vi "LS218_INIT_VOIES.vi"(2 "Tableau 2":T1(array[cluster]), 7 "entrée d'erreur (pas d'erreur)":errorcluster, 10 "Refnum VISA en entrée":refnum<visa-resource-name>) -> (0 "error out":errorcluster, 3 "Refnum VISA en entrée 2":refnum<visa-resource-name>)   [LabVIEW 2014]
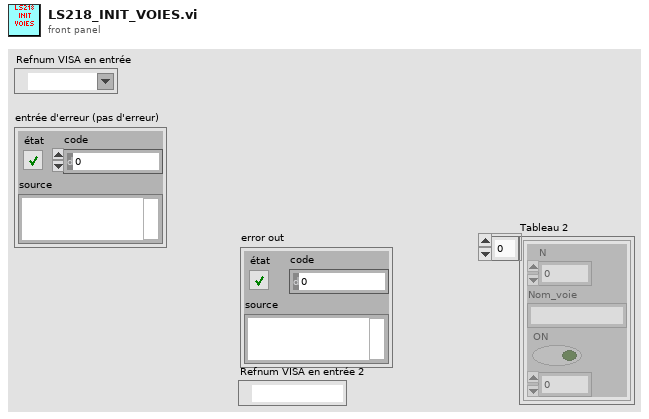
[diagram p1: front panel]
types:
  T1 = cluster{"N":i32, "Nom_voie":string, "ON":bool, dbl}[]
  T2 = cluster{"N":i32, "Nom_voie":string, "ON":bool, dbl}
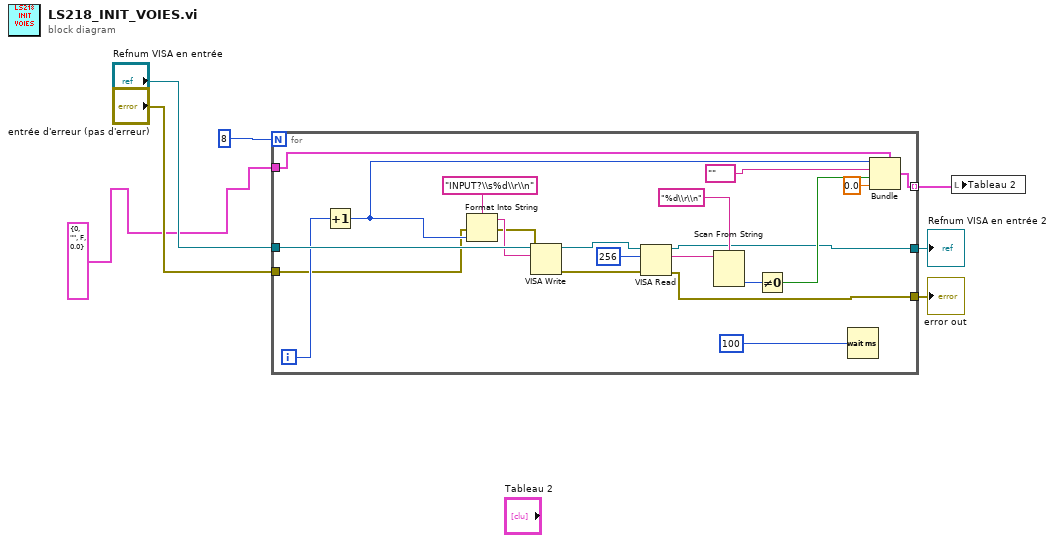
[diagram p0: block diagram]
diagram:
  n1 = for {
    N: 8 -> [_]
    tunnel: "Refnum VISA en entrée" -> [w26]
    tunnel: "entrée d'erreur (pas d'erreur)" -> [w9]
    tunnel: T2 {"N"=0, "Nom_voie"="", "ON"=FALSE, 0.0} ("Voies de mesure") -> [w17]
    tunnel: [w12] -> w1 mode=indexing
    tunnel: [w11] -> w4
    tunnel: [w10] -> w3
    i -> [w18]
    n2 = Increment(x=w18) -> (x+1=w16:i32)
    n3 = Format Into String(format string="INPUT?\\s%d\\r\\n" ("chaîne de format"), error in=w9, w16) -> (resulting string=w19:string, error out=w8:errorcluster)  [unwired: 1 in]
    n4 = VISA Write(VISA resource name=w26, write buffer=w19, error in (no error)=w8) -> (VISA resource name out=w24:refnum<visa-resource-name>, error out=w23:errorcluster)  [unwired: 1 out]
    n5 = VISA Read(VISA resource name=w24, byte count=u32 256 ("nombre d'octets"), error in (no error)=w23) -> (VISA resource name out=w10:refnum<visa-resource-name>, read buffer=w21:string, error out=w11:errorcluster)  [unwired: 1 out]
    n6 = Scan From String(format string="%d\\r\\n" ("chaîne de format"), input string=w21) -> (output 1=w20:i32)  [unwired: 3 in, 3 out]
    n7 = Not Equal To 0?(x=w20) -> (x != 0?=w14:bool)
    n8 = Wait (ms)(milliseconds to wait=u32 100 ("attente (ms)")) -> ()  [unwired: 1 out]
    n9 = Bundle(cluster=w17, "N"=w16, "Nom_voie"="", "ON"=w14, 0.0) -> (w12:T2)
  }
  "error out" <- w4
  "Refnum VISA en entrée 2" <- w3
  n10 = local write "Tableau 2"(w1) -> ()
